vi "Usermgt.vi"(8 "error In":errorcluster) -> (0 "error out":errorcluster)   [LabVIEW 2015]
uses:
  Um- Save.ctl
  Um-Delete.ctl
  Um-Exit.ctl
  <vilib>/addons/database/Connection.llb/DB Tools Open Connec (String).vi
  <vilib>/addons/database/_DB Variant To Data/Database Variant To Data.xnode
  <vilib>/addons/database/NI_Database_API.lvlib
panel:
  in  "Operator ID":string
  out "User Name 2":string
  out "error out 2":errorcluster
  in  "Exit":T1
  in  "Deleat":T2
  in  "Save":T3
  in  "User Type":string
  in  "User Type":u16(ring) items=["Operator", "Supervisor", "admin"]
  in  "Re-Password":string
  in  "Password":string
  in  "User Name":string
  in  "User Table":i32(listbox)
  # "User Create"
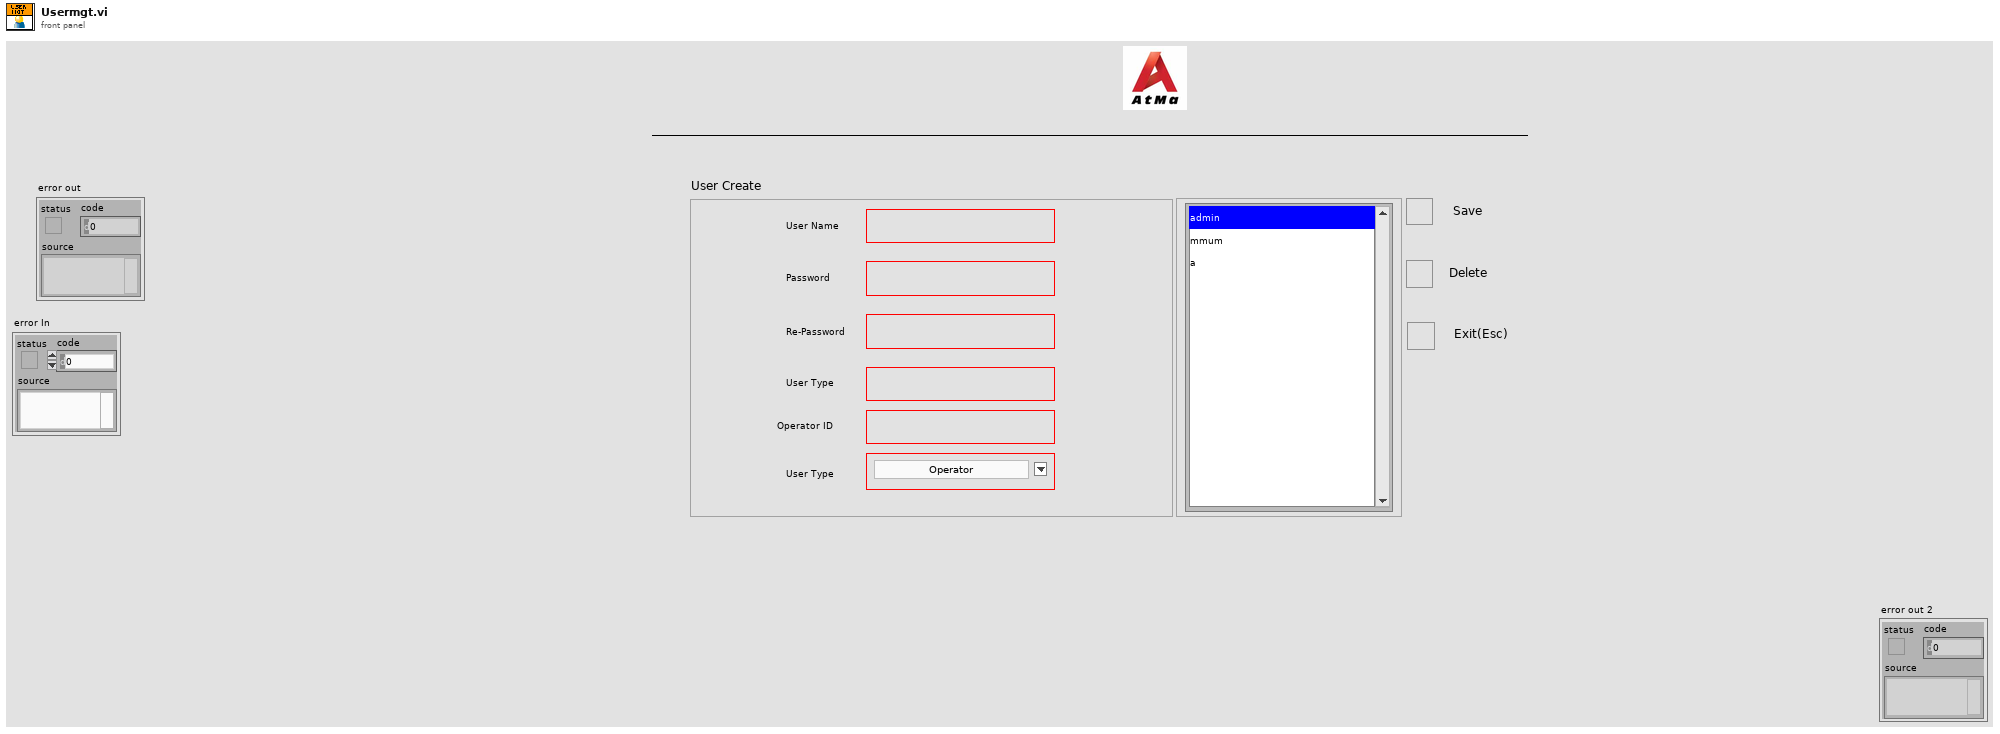
[diagram p1: front panel]
types:
  T1 = typedef "Um-Exit.ctl" = bool
  T2 = typedef "Um-Delete.ctl" = bool
  T3 = typedef "Um- Save.ctl" = bool
  T4 = cluster{"User Name":string, "Password":string, "User Type":string}
  T5 = typedef "NI_Database_API.lvlib/Conn ObjectReference.ctl" = refnum<k1>
  T6 = cluster{"User Name":string, "Password":string, "User Type":string, "Access right":string}
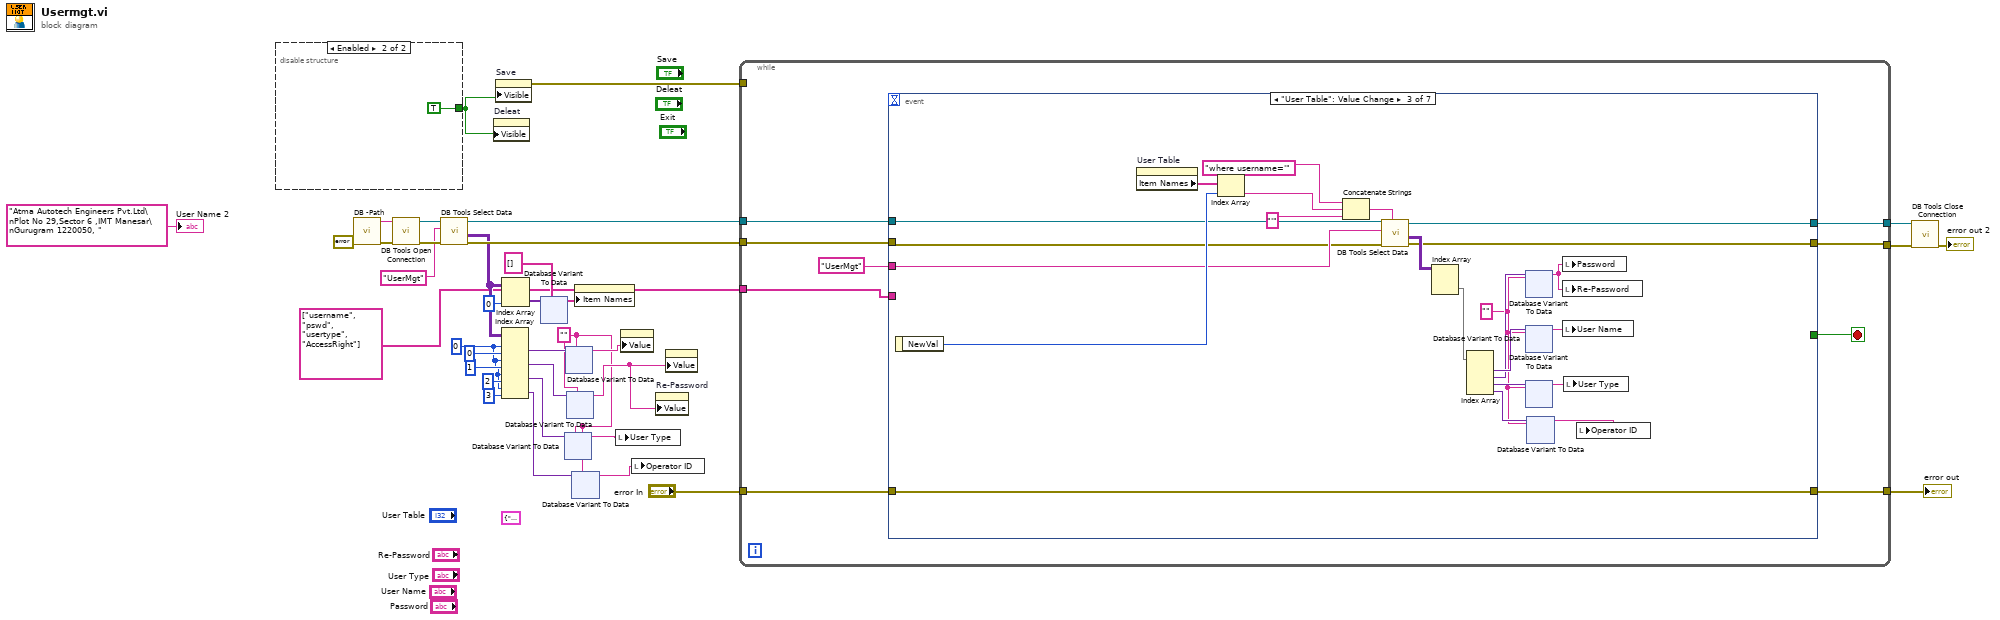
[diagram p0: block diagram]
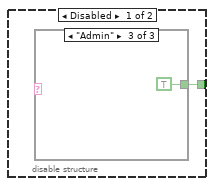
[diagram p2: hidden frame]
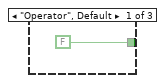
[diagram p3: hidden frame]
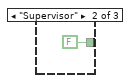
[diagram p4: hidden frame]
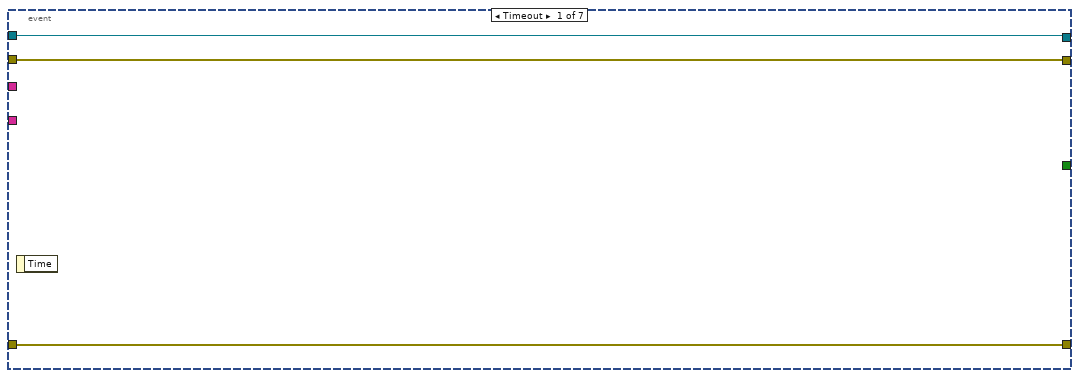
[diagram p5: hidden frame]
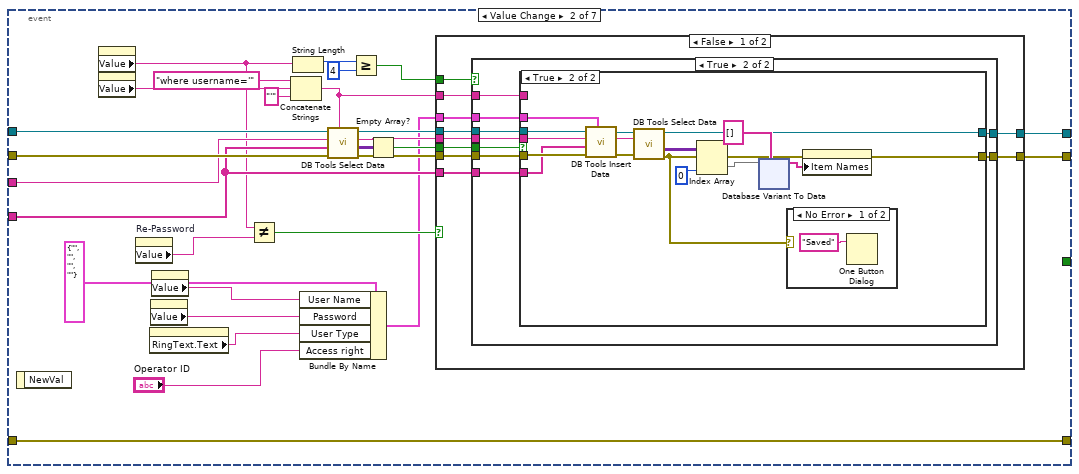
[diagram p6: hidden frame]
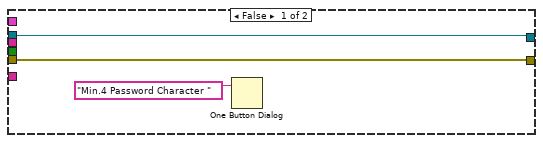
[diagram p7: hidden frame]
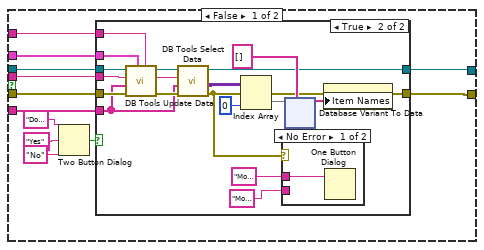
[diagram p8: hidden frame]
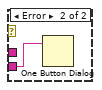
[diagram p10: hidden frame]
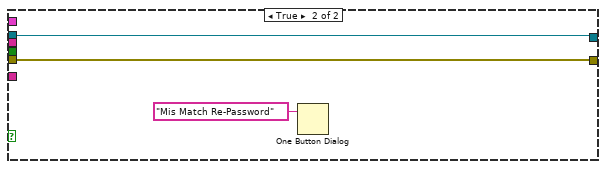
[diagram p12: hidden frame]
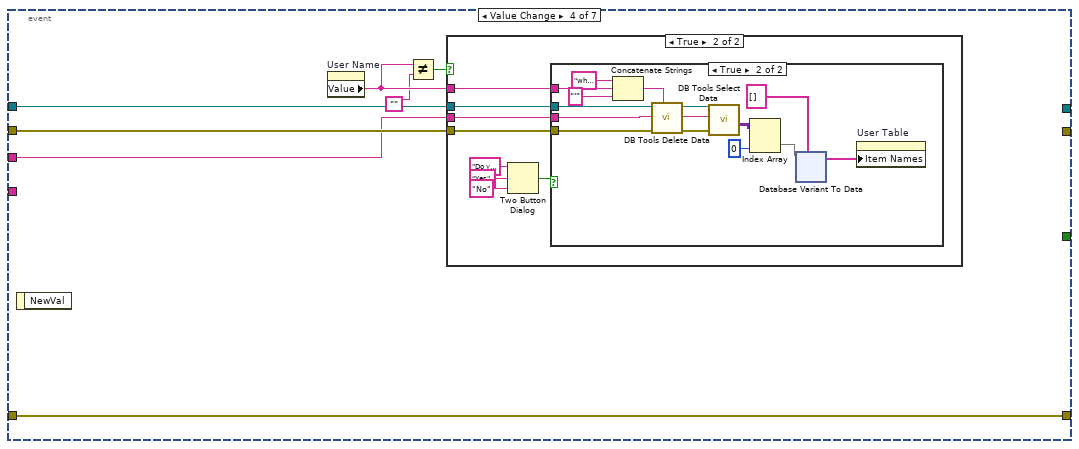
[diagram p13: hidden frame]
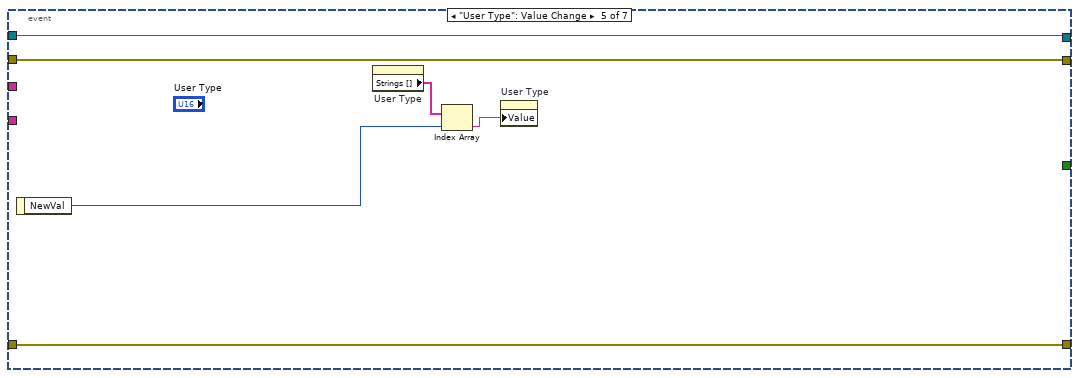
[diagram p16: hidden frame]
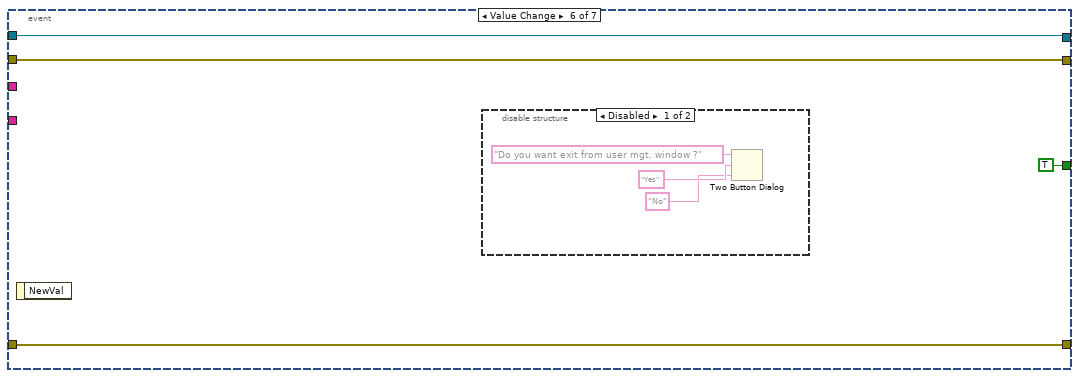
[diagram p17: hidden frame]
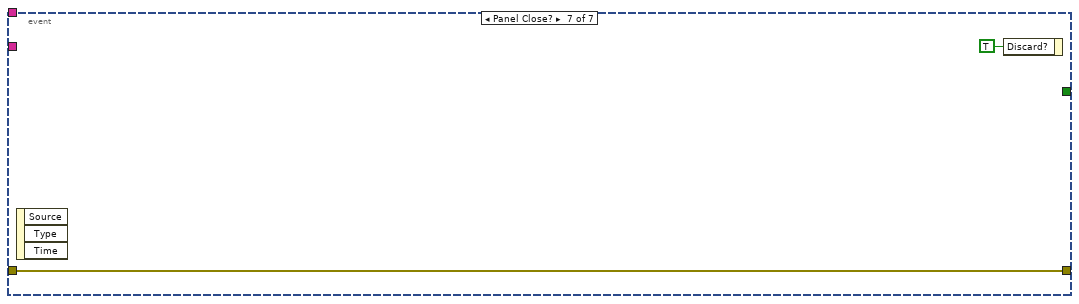
[diagram p19: hidden frame]
diagram:
  w5 = ""
  w3 = 0 ("index (row)")
  (unwired) T4 {"User Name"="", "Password"="", "User Type"=""} ("Input data")
  n1 = disable-structure shown="Enabled" {
    disable-tunnel: [w36 TRUE] -> w13
    frame Disabled {
      n2 = case shown="\"Admin\"" {
        selector: _ -> [_ _ _]
        tunnel: [FALSE FALSE TRUE] -> w36
        frame "Operator", Default {
        }
        frame "Supervisor" {
        }
        frame "Admin" {
        }
      }
    }
    frame Enabled {
    }
  }
  n3 = call "DB -Path.vi"() -> ("String"=w35:string)  [unwired: 11 in]
  n4 = call-poly <vilib>:"DB Tools Open Connection.vi"("error in (no error)"=errorcluster {"status"=FALSE, "code"=0, "source"=""}, "connection information"=w35) -> ("error out"=w32:errorcluster, "connection reference"=w31:T5)  [unwired: 6 in]
  n5 = call <vilib>:"DB Tools Select Data.vi"("error in (no error)"=w32, "table"="UserMgt", "connection reference"=w31) -> ("error out"=w29:errorcluster, "data"=w22:variant[][], "connection reference out"=w30:T5)  [unwired: 3 in]
  n6 = property on="Deleat" class="Bool (strict)"("Visible"=w13) -> ()  [unwired: 2 in, 2 out]
  n7 = property on="Save" class="Bool (strict)"("Visible"=w13) -> (error out=w12:errorcluster)  [unwired: 2 in, 1 out]
  n8 = Index Array(array=w22, index (row) #1=w3, index (col) #1=0 ("disabled index (col)"), index (row) #2=w3, index (col) #2=1 ("disabled index (col)"), index (row) #3=w3, index (col) #3=2 ("disabled index (col)"), index (row) #4=w3, index (col) #4=3 ("index (col)")) -> (element #1=w23:variant, element #2=w19:variant, element #3=w15:variant, element #4=w2:variant)
  n9 = Index Array(array=w22, index (col)=0 ("disabled index (col)")) -> (element=w27:variant[])  [unwired: 1 in]
  n10 = xnode "Database Variant To Data"("database variant"=w27, "type"=string[] []) -> ("data"=w24:string[])  [unwired: 1 in, 1 out]
  n11 = xnode "Database Variant To Data"("database variant"=w15, "type"=w5) -> ("data"=w14:string)  [unwired: 1 in, 1 out]
  n12 = xnode "Database Variant To Data"("database variant"=w23, "type"=w5) -> ("data"=w18:string)  [unwired: 1 in, 1 out]
  n13 = xnode "Database Variant To Data"("database variant"=w19, "type"=w5) -> ("data"=w17:string)  [unwired: 1 in, 1 out]
  n14 = xnode "Database Variant To Data"("database variant"=w2, "type"=w5) -> ("data"=w1:string)  [unwired: 1 in, 1 out]
  n15 = property on="User Table" class="LstBox (strict)"("Item Names"=w24) -> ()  [unwired: 2 in, 2 out]
  n16 = local write "User Type"(w14) -> ()
  n17 = property on="User Name" class="Str"("Value"=w18) -> ()  [unwired: 2 in, 2 out]
  n18 = local write "Operator ID"(w1) -> ()
  n19 = property on="Re-Password" class="Str"("Value"=w17) -> ()  [unwired: 2 in, 2 out]
  n20 = property on="Password" class="Str"("Value"=w17) -> ()  [unwired: 2 in, 2 out]
  n21 = while {
    tunnel: w30 -> [w48]
    tunnel: w29 -> [w47]
    tunnel: [w45] -> w34
    tunnel: [w44] -> w33
    tunnel: w12 -> [_]
    tunnel: string[] ["username", "pswd", "usertype", "AccessRight"] ("columns") -> [w43]
    tunnel: "error In" -> [w42]
    tunnel: [w41] -> w8
    stop <- w49 stop-if-true
    n22 = event shown="[2] \"User Table\": Value Change" {
      selector: _ -> [_ _ _ _ _ _ _]
      dyn-events: _ -> [_ _ _ _ _ _ _]
      timeout: _ -> [_ _ _ _ _ _ _]
      tunnel: [_ _ _ _ _ TRUE ("T button?") _] -> w49
      tunnel: w48 -> [w52 w79 w237 w386 w449 w456 _]
      tunnel: w47 -> [w51 w78 w236 w385 w448 w455 _]
      tunnel: "UserMgt" ("table") -> [_ w71 w245 w381 _ _ _]
      tunnel: w43 -> [_ w70 _ _ _ _ _]
      tunnel: [w52 w69 w235 _ w449 w456 _] -> w45
      tunnel: [w51 w68 w234 _ w448 w455 _] -> w44
      tunnel: w42 -> [w50 w54 w232 w380 w447 w453 w460]
      tunnel: [w50 w54 w232 w380 w447 w453 w460] -> w41
      event Timeout {
        n23 = event-data() -> ()  [unwired: 1 in, 1 out]
      }
      event Value Change {
        n24 = event-data() -> ()  [unwired: 1 in, 1 out]
        n25 = property on="Password" class="Str"() -> ("Value"=w56:string)  [unwired: 2 in, 2 out]
        n26 = property on="User Name" class="Str"() -> ("Value"=w55:string)  [unwired: 2 in, 2 out]
        n27 = property on="Re-Password" class="Str"() -> ("Value"=w62:string)  [unwired: 2 in, 2 out]
        n28 = property on="User Type" class="Ring (strict)"() -> ("RingText.Text"=w59:string)  [unwired: 2 in, 2 out]
        n29 = property on="Password" class="Str"() -> ("Value"=w61:string)  [unwired: 2 in, 2 out]
        n30 = property on="User Name" class="Str"() -> ("Value"=w60:string)  [unwired: 2 in, 2 out]
        n31 = Not Equal?(x=w56, y=w62) -> (x != y?=w63:bool)
        n32 = Concatenate Strings("where username='" ("condition"), w55, "'" ("User Name")) -> (w67:string)
        n33 = String Length(string=w56) -> (length=w66:i32)
        n34 = Bundle By Name(cluster=T6 {"User Name"="", "Password"="", "User Type"="", "Access right"=""} ("input cluster"), "User Name"=w60, "Password"=w61, "User Type"=w59, "Access right"="Operator ID") -> (w57:T6)
        n35 = call <vilib>:"DB Tools Select Data.vi"("condition"=w67, "error in (no error)"=w78, "columns"=w70, "table"=w71, "connection reference"=w79) -> ("error out"=w72:errorcluster, "data"=w77:variant[][], "connection reference out"=w73:T5)  [unwired: 1 in]
        n36 = Greater Or Equal?(x=w66, y=4) -> (x >= y?=w64:bool)
        n37 = Empty Array?(array=w77) -> (empty?=w76:bool)
        n38 = case shown="False" w63 {
          tunnel: w76 -> [w89 _]
          tunnel: w73 -> [w88 w228]
          tunnel: w72 -> [w87 w227]
          tunnel: w71 -> [w86 _]
          tunnel: w70 -> [w85 _]
          tunnel: w57 -> [w84 _]
          tunnel: [w83 w228] -> w69
          tunnel: [w82 w227] -> w68
          tunnel: w67 -> [w81 _]
          tunnel: w64 -> [w80 _]
          frame False {
            n39 = case shown="True" w80 {
              tunnel: w89 -> [_ w101]
              tunnel: w88 -> [w92 w100]
              tunnel: w87 -> [w91 w99]
              tunnel: w86 -> [_ w98]
              tunnel: w85 -> [_ w97]
              tunnel: w84 -> [_ w96]
              tunnel: [w92 w95] -> w83
              tunnel: [w91 w94] -> w82
              tunnel: w81 -> [_ w93]
              frame False {
                n40 = One Button Dialog(message="Min.4 Password Character ") -> ()  [unwired: 1 in, 1 out]
              }
              frame True {
                n41 = case shown="True" w101 {
                  tunnel: w100 -> [w113 w186]
                  tunnel: w99 -> [w112 w185]
                  tunnel: w98 -> [w107 w180]
                  tunnel: w97 -> [w104 w184]
                  tunnel: w96 -> [w105 w183]
                  tunnel: [w103 w174] -> w95
                  tunnel: [w102 w173] -> w94
                  tunnel: w93 -> [w106 _]
                  frame False {
                    n42 = Two Button Dialog(message="Do you want  modification" ("T button name (\"OK\")"), 1:"No" ("F button name (\"Cancel\")"), 2:"Yes" ("T button name (\"OK\")")) -> (T button?=w111:bool)
                    n43 = case shown="True" w111 {
                      tunnel: w113 -> [w115 w132]
                      tunnel: w112 -> [w114 w131]
                      tunnel: w107 -> [_ w126]
                      tunnel: w106 -> [_ w130]
                      tunnel: w105 -> [_ w129]
                      tunnel: w104 -> [_ w120]
                      tunnel: [w115 w119] -> w103
                      tunnel: [w114 w118] -> w102
                      frame False {
                      }
                      frame True {
                        n44 = call <vilib>:"DB Tools Update Data.vi"("condition"=w130, "data"=w129, "error in (no error)"=w131, "columns"=w120, "table"=w126, "connection reference"=w132) -> ("error out"=w127:errorcluster, "connection reference out"=w128:T5)  [unwired: 4 in]
                        n45 = call <vilib>:"DB Tools Select Data.vi"("error in (no error)"=w127, "columns"=w120, "table"=w126, "connection reference"=w128) -> ("error out"=w118:errorcluster, "data"=w125:variant[][], "connection reference out"=w119:T5)  [unwired: 2 in]
                        n46 = Index Array(array=w125, index (col)=0 ("disabled index (col)")) -> (element=w123:variant[])  [unwired: 1 in]
                        n47 = case shown="No Error" w118 {
                          tunnel: "Modification is Successfully" ("T button name (\"OK\")") -> [w133 _]
                          tunnel: "Modification is Unsuccessfully" ("T button name (\"OK\")") -> [_ w134]
                          frame No Error {
                            n48 = One Button Dialog(message=w133) -> ()  [unwired: 1 in, 1 out]
                          }
                          frame Error {
                            n49 = One Button Dialog(message=w134) -> ()  [unwired: 1 in, 1 out]
                          }
                        }
                        n50 = xnode "Database Variant To Data"("database variant"=w123, "type"=string[] []) -> ("data"=w121:string[])  [unwired: 1 in, 1 out]
                        n51 = property on="User Table" class="LstBox (strict)"("Item Names"=w121) -> ()  [unwired: 2 in, 2 out]
                      }
                    }
                  }
                  frame True {
                    n52 = call <vilib>:"DB Tools Insert Data.vi"("data"=w183, "error in (no error)"=w185, "columns"=w184, "table"=w180, "connection reference"=w186) -> ("error out"=w181:errorcluster, "connection reference out"=w182:T5)  [unwired: 5 in]
                    n53 = call <vilib>:"DB Tools Select Data.vi"("error in (no error)"=w181, "table"=w180, "connection reference"=w182) -> ("error out"=w173:errorcluster, "data"=w179:variant[][], "connection reference out"=w174:T5)  [unwired: 3 in]
                    n54 = Index Array(array=w179, index (col)=0 ("disabled index (col)")) -> (element=w177:variant[])  [unwired: 1 in]
                    n55 = xnode "Database Variant To Data"("database variant"=w177, "type"=string[] []) -> ("data"=w175:string[])  [unwired: 1 in, 1 out]
                    n56 = case shown="No Error" w173 {
                      frame No Error {
                        n57 = One Button Dialog(message="Saved" ("T button name (\"OK\")")) -> ()  [unwired: 1 in, 1 out]
                      }
                      frame Error {
                      }
                    }
                    n58 = property on="User Table" class="LstBox (strict)"("Item Names"=w175) -> ()  [unwired: 2 in, 2 out]
                  }
                }
              }
            }
          }
          frame True {
            n59 = One Button Dialog(message="Mis Match Re-Password") -> ()  [unwired: 1 in, 1 out]
          }
        }
      }
      event "User Table": Value Change {
        w230 = "" ("table")
        n60 = event-data() -> ("NewVal"=w249:i32)  [unwired: 1 in]
        n61 = property on="User Table" class="LstBox (strict)"() -> ("Item Names"=w250:string[])  [unwired: 2 in, 2 out]
        n62 = Index Array(array=w250, index=w249) -> (element=w247:string)
        n63 = Concatenate Strings("where username='" ("condition"), w247, "'" ("User Name")) -> (w246:string)
        n64 = call <vilib>:"DB Tools Select Data.vi"("condition"=w246, "error in (no error)"=w236, "table"=w245, "connection reference"=w237) -> ("error out"=w234:errorcluster, "data"=w244:variant[][], "connection reference out"=w235:T5)  [unwired: 2 in]
        n65 = Index Array(array=w244) -> (element=w243:variant[])  [unwired: 2 in]
        n66 = Index Array(array=w243) -> (element #1=w242:variant, element #2=w241:variant, element #3=w240:variant, element #4=w231:variant)  [unwired: 4 in]
        n67 = xnode "Database Variant To Data"("database variant"=w241, "type"=w230) -> ("data"=w238:string)  [unwired: 1 in, 1 out]
        n68 = xnode "Database Variant To Data"("database variant"=w242, "type"=w230) -> ("data"=w239:string)  [unwired: 1 in, 1 out]
        n69 = xnode "Database Variant To Data"("database variant"=w240, "type"=w230) -> ("data"=w233:string)  [unwired: 1 in, 1 out]
        n70 = xnode "Database Variant To Data"("database variant"=w231, "type"=w230) -> ("data"=w229:string)  [unwired: 1 in, 1 out]
        n71 = local write "Password"(w238) -> ()
        n72 = local write "Re-Password"(w238) -> ()
        n73 = local write "User Name"(w239) -> ()
        n74 = local write "User Type"(w233) -> ()
        n75 = local write "Operator ID"(w229) -> ()
      }
      event Value Change {
        n76 = event-data() -> ()  [unwired: 1 in, 1 out]
        n77 = property on="User Name" class="Str"() -> ("Value"=w384:string)  [unwired: 2 in, 2 out]
        n78 = Not Equal?(x=w384, y="") -> (x != y?=w382:bool)
        n79 = case shown="True" w382 {
          tunnel: w386 -> [_ w390]
          tunnel: w385 -> [_ w389]
          tunnel: w384 -> [_ w388]
          tunnel: w381 -> [_ w387]
          frame False {
          }
          frame True {
            n80 = Two Button Dialog(message="Do you want delete the user id & password", 1:"No" ("F button name (\"Cancel\")"), 2:"Yes" ("T button name (\"OK\")")) -> (T button?=w391:bool)
            n81 = case shown="True" w391 {
              tunnel: w390 -> [_ w408]
              tunnel: w389 -> [_ w407]
              tunnel: w388 -> [_ w403]
              tunnel: w387 -> [_ w400]
              frame False {
              }
              frame True {
                n82 = Concatenate Strings("where username='" ("condition"), w403, "'" ("User Name")) -> (w404:string)
                n83 = call <vilib>:"DB Tools Delete Data.vi"("condition"=w404, "error in (no error)"=w407, "table"=w400, "connection reference"=w408) -> ("error out"=w401:errorcluster, "connection reference out"=w402:T5)  [unwired: 6 in]
                n84 = call <vilib>:"DB Tools Select Data.vi"("error in (no error)"=w401, "table"=w400, "connection reference"=w402) -> ("data"=w398:variant[][])  [unwired: 3 in, 2 out]
                n85 = Index Array(array=w398, index (col)=0 ("disabled index (col)")) -> (element=w397:variant[])  [unwired: 1 in]
                n86 = xnode "Database Variant To Data"("database variant"=w397, "type"=string[] []) -> ("data"=w395:string[])  [unwired: 1 in, 1 out]
                n87 = property on="User Table" class="LstBox (strict)"("Item Names"=w395) -> ()  [unwired: 2 in, 2 out]
              }
            }
          }
        }
      }
      event "User Type": Value Change {
        n88 = event-data() -> ("NewVal"=w452:u16)  [unwired: 1 in]
        n89 = property on="User Type" class="Ring (strict)"() -> ("Strings []"=w451:string[])  [unwired: 2 in, 2 out]
        n90 = Index Array(array=w451, index=w452) -> (element=w450:string)
        n91 = property on="User Type" class="Str"("Value"=w450) -> ()  [unwired: 2 in, 2 out]
      }
      event Value Change {
        n92 = event-data() -> ()  [unwired: 1 in, 1 out]
        n93 = disable-structure shown="Disabled" {
          frame Disabled {
            n94 = Two Button Dialog(message="Do you want exit from user mgt. window ?", 1:"No" ("F button name (\"Cancel\")"), 2:"Yes" ("T button name (\"OK\")")) -> ()  [unwired: 1 out]
          }
          frame Enabled {
          }
        }
      }
      event Panel Close? {
        n95 = event-data() -> ()  [unwired: 1 in, 3 out]
        n96 = event-data("Discard?"=TRUE) -> ()  [unwired: 1 in, 1 out]
      }
    }
  }
  "error out" <- w8
  n97 = call <vilib>:"DB Tools Close Connection.vi"("error in (no error)"=w33, "connection reference"=w34) -> ("error out"=→"error out 2":errorcluster)  [unwired: 5 in]
  "User Name 2" <- "Atma Autotech Engineers Pvt.Ltd\nPlot No 29,Sector 6 ,IMT Manesar\nGurugram 1220050, " ("string")
